vi "数据结构1.vi"() -> ()   [LabVIEW 2017]
panel:
  in  "布尔":bool
  out "数值 3":dbl
  in  "下拉列表":u16(ring) items=["AA"=100, "BB"=33, "CC"=22]
  out "字符串 3":string
  out "字符串 2":string
  out "字符串":string
  in  "枚举":enum16{"AA", "BB", "CC"}(ring)
  out "x+y":u32
  in  "数值 2":u32
  in  "数值":u32
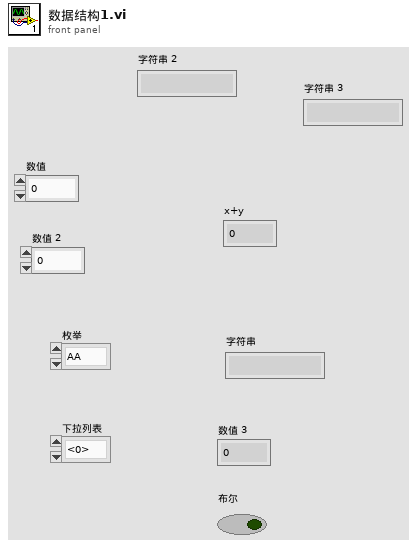
[diagram p1: front panel]
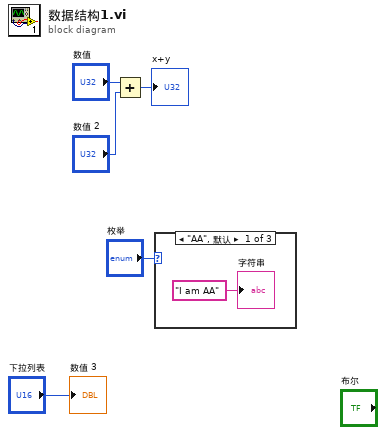
[diagram p0: block diagram]
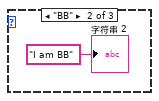
[diagram p2: hidden frame]
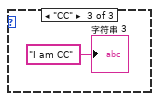
[diagram p3: hidden frame]
diagram:
  n1 = Add(x="数值", y="数值 2") -> (x+y=→"x+y":u32)
  n2 = case shown="\"AA\", 默认" "枚举" {
    frame "AA", Default {
      "字符串" <- "I am AA" ("字符串")
    }
    frame "BB" {
      "字符串 2" <- "I am BB" ("字符串 2")
    }
    frame "CC" {
      "字符串 3" <- "I am CC" ("字符串 2")
    }
  }
  "数值 3" <- "下拉列表"
